vi "Include Default Region in URL.vi"(11 "AWS Core":refnum<class "HTTP Request.lvclass">) -> (3 "Include Default Region":bool)   [LabVIEW 2015, in "NI_AWS_Core.lvlib" / "HTTP Request.lvclass"]
uses:
  HTTP Request.lvclass
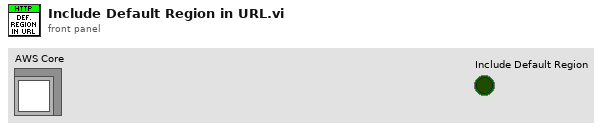
[diagram p1: front panel]
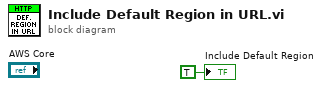
[diagram p0: block diagram]
diagram:
  "Include Default Region" <- TRUE ("Include Default Region")
